vi "Power ON_OFF.vi"(8 "error in (no error)":errorcluster, 10 "Power":bool, 11 "DAQ HVPS in":refnum<class "DAQ HVPS.lvclass">) -> (0 "error out":errorcluster, 3 "DAQ HVPS out":refnum<class "DAQ HVPS.lvclass">)   [LabVIEW 2014, in "DAQ HVPS.lvclass"]
uses:
  DAQ HVPS.lvclass
  DAQ HVPS.lvclass/DAQ HVPS.ctl
  <vilib>/DAQmx/write.llb/DAQmx Write (Digital Bool 1Line 1Point).vi
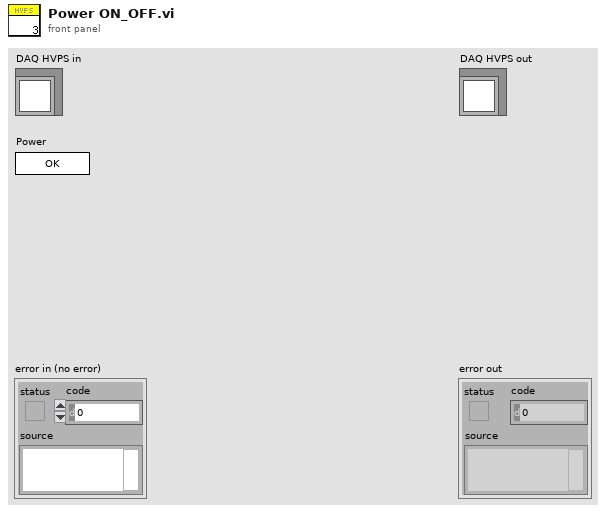
[diagram p1: front panel]
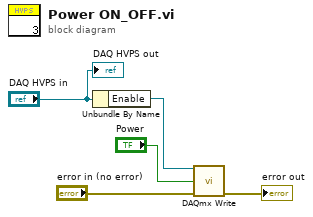
[diagram p0: block diagram]
diagram:
  n1 = Unbundle By Name("DAQ HVPS in") -> ("Enable"=w3:refnum<k21>)
  n2 = call-poly <vilib>:"DAQmx Write.vi"("task/channels in"=w3, "data"="Power", "error in"="error in (no error)") -> ("error out"=→"error out":errorcluster)  [unwired: 10 in, 2 out]
  "DAQ HVPS out" <- "DAQ HVPS in"
